vi "Ctor.vi"(6 "Name (Caller VI)":string, 8 "error in (no error)":errorcluster) -> (0 "error out":errorcluster, 3 "PanelArray":refnum<class "ArrayManager.lvclass">)   [LabVIEW 2020, in "OOPanel.lvlib" / "ArrayManager.lvclass"]
uses:
  ArrayManager.lvclass
  ArrayPanel/ArrayPanel.lvclass
  UI Refs.ctl
  Events.ctl
  State Ref.ctl
  Event Regs.ctl
  ArrayManager.lvclass/ArrayManager.ctl
  Manager/Manager.lvclass
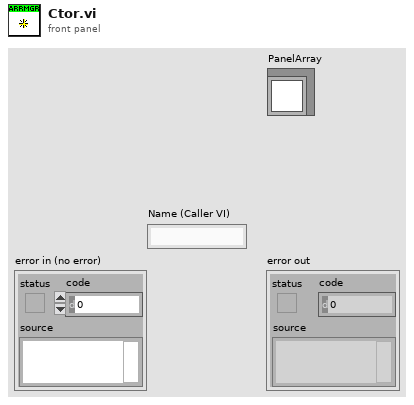
[diagram p1: front panel]
types:
  T1 = typedef "OOPanel.lvlib/ArrayManager.lvclass/Event Regs.ctl" = cluster{"Event Reg":refnum<event-registration>, "Last Update Ticks ms":u32}
  T2 = typedef "OOPanel.lvlib/ArrayManager.lvclass/State Ref.ctl" = cluster{"Running":bool, "Borders":bool, "Total Height":dbl, "Scroll Visible":bool}
  T3 = typedef "OOPanel.lvlib/ArrayManager.lvclass/Events.ctl" = cluster{"Stop":refnum<user-event>, "Update":refnum<user-event>, "Scroll":refnum<user-event>}
  T4 = typedef "OOPanel.lvlib/ArrayManager.lvclass/UI Refs.ctl" = cluster{"SubPanels":refnum<vi>[], "Scrollbar":refnum<vi>, "Panel VI":refnum<vi>, "Container":refnum<vi>}
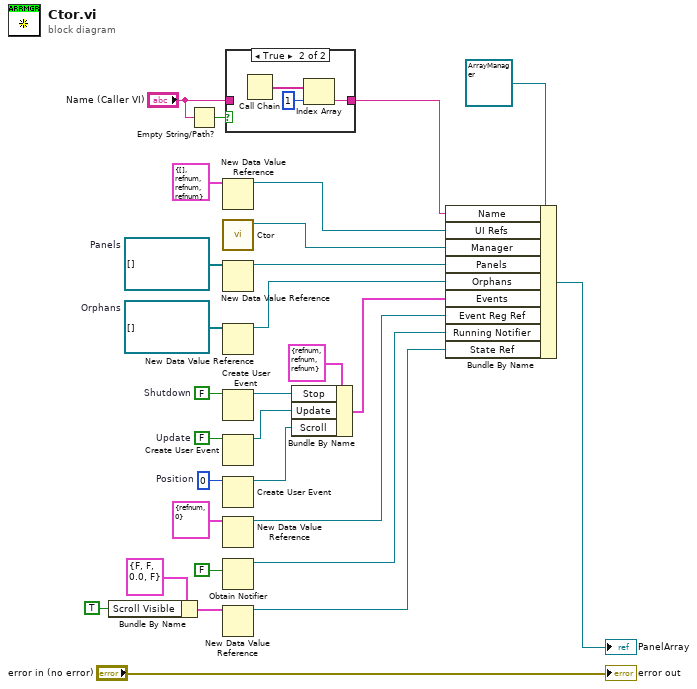
[diagram p0: block diagram]
diagram:
  w8 = 0  # Position
  w16 = FALSE  # Update
  w22 = refnum<class "ArrayPanel.lvclass">[] []  # Orphans
  w23 = refnum<class "ArrayPanel.lvclass">[] []  # Panels
  w25 = FALSE  # Shutdown
  n1 = Bundle By Name(cluster=T2 {"Running"=FALSE, "Borders"=FALSE, "Total Height"=0.0, "Scroll Visible"=FALSE} ("State Ref"), "Scroll Visible"=TRUE) -> (w10:T2)
  n2 = Empty String/Path?(string/path="Name (Caller VI)") -> (empty?=w3:bool)
  n3 = New Data Value Reference(data value=T4 {"SubPanels"=[], "Scrollbar"=refnum, "Panel VI"=refnum, "Container"=refnum} ("UI Refs")) -> (data value reference=w18:refnum<data-value>)  [unwired: 1 in, 1 out]
  n4 = call "Ctor.vi"() -> ("Manager out"=w26:refnum<class "Manager.lvclass">)  [unwired: 10 in, 1 out]
  n5 = New Data Value Reference(data value=w23) -> (data value reference=w21:refnum<data-value>)  [unwired: 1 in, 1 out]
  n6 = New Data Value Reference(data value=w22) -> (data value reference=w20:refnum<data-value>)  [unwired: 1 in, 1 out]
  n7 = Create User Event(user event datatype=w25) -> (user event=w24:refnum<user-event>)  [unwired: 1 in, 1 out]
  n8 = Create User Event(user event datatype=w16) -> (user event=w15:refnum<user-event>)  [unwired: 1 in, 1 out]
  n9 = Create User Event(user event datatype=w8) -> (user event=w7:refnum<user-event>)  [unwired: 1 in, 1 out]
  n10 = New Data Value Reference(data value=T1 {"Event Reg"=refnum, "Last Update Ticks ms"=0} ("Event Reg State")) -> (data value reference=w4:refnum<data-value>)  [unwired: 1 in, 1 out]
  n11 = Obtain Notifier(notification data type=FALSE) -> (notifier out=w13:refnum<notifier>)  [unwired: 3 in, 2 out]
  n12 = New Data Value Reference(data value=w10) -> (data value reference=w11:refnum<data-value>)  [unwired: 1 in, 1 out]
  n13 = case shown="True" w3 {
    tunnel: "Name (Caller VI)" -> [w30 _]
    tunnel: [w30 w31] -> w1
    frame False {
    }
    frame True {
      n14 = Call Chain() -> (call chain=w33:string[])
      n15 = Index Array(array=w33, index=1) -> (element=w31:string)
    }
  }
  n16 = Bundle By Name(cluster=T3 {"Stop"=refnum, "Update"=refnum, "Scroll"=refnum} ("Events"), "Stop"=w24, "Update"=w15, "Scroll"=w7) -> (w6:T3)
  n17 = Bundle By Name(cluster=refnum<class "ArrayManager.lvclass"> refnum ("PanelArray in"), "Name"=w1, "UI Refs"=w18, "Manager"=w26, "Panels"=w21, "Orphans"=w20, "Events"=w6, "Event Reg Ref"=w4, "Running Notifier"=w13, "State Ref"=w11) -> (→"PanelArray":refnum<class "ArrayManager.lvclass">)
  "error out" <- "error in (no error)"
